vi "Test Symmetric (CDB).vi"(9 "relative tolerance?":bool, 10 "tolerance":dbl=-1.0, 11 "Input Matrix":T1) -> (0 "error":i32, 3 "Symmetric?":bool)   [LabVIEW 2020, in "NI_AALPro.lvlib"]
uses:
  <vilib>/Analysis/NI_AALPro.lvlib
  <vilib>/Analysis/Matrix/Datatypes/ComplexMatrix.ctl
  <resource>/lvanlys.dll
  <vilib>/Analysis/Matrix/NI_Matrix.lvlib
panel:
  # "Test Symmetric"
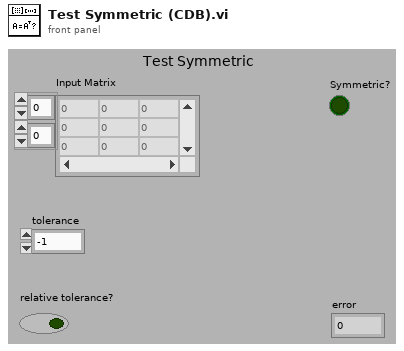
[diagram p1: front panel]
types:
  T1 = typedef "NI_Matrix.lvlib/ComplexMatrix.ctl" = cdb[][]
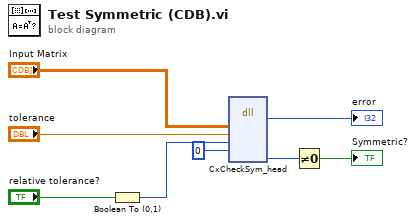
[diagram p0: block diagram]
diagram:
  n1 = Boolean To (0,1)(Boolean="relative tolerance?") -> (0, 1=w5:i16)
  n2 = dll-call lib="e:/builds/penguin/labview/branches/2020/dev/dist/resource/lvanlys.*" fn="CxCheckSym_head" ("lvanlys.dll:CxCheckPosSemiDef_head")("_aH"="Input Matrix", "_tol"="tolerance", "_reltol"=w5, "_conj"=0) -> ("return type"=→"error":i32, "_sym"=w4:i32)  [unwired: 6 in, 4 out]
  n3 = Not Equal To 0?(x=w4) -> (x != 0?=→"Symmetric?":bool)
